vi "VI Tree.vi"   [LabVIEW 2022 SP3, in "Agilent ENA Series.lvlib"]
doc: "This is the instrument driver for the Agilent ENA Series RF Network Analyzer. The VI Tree displays all the user-callable VIs of the instrument driver in an organized table."
uses:
  <instrlib>/Agilent ENA Series/Agilent ENA Series.lvlib
panel:
  # "(c) 2005-2021 National Instruments.  ALL RIGHTS RESERVED."
  # "SEE DIAGRAM\nFOR VI TREE."
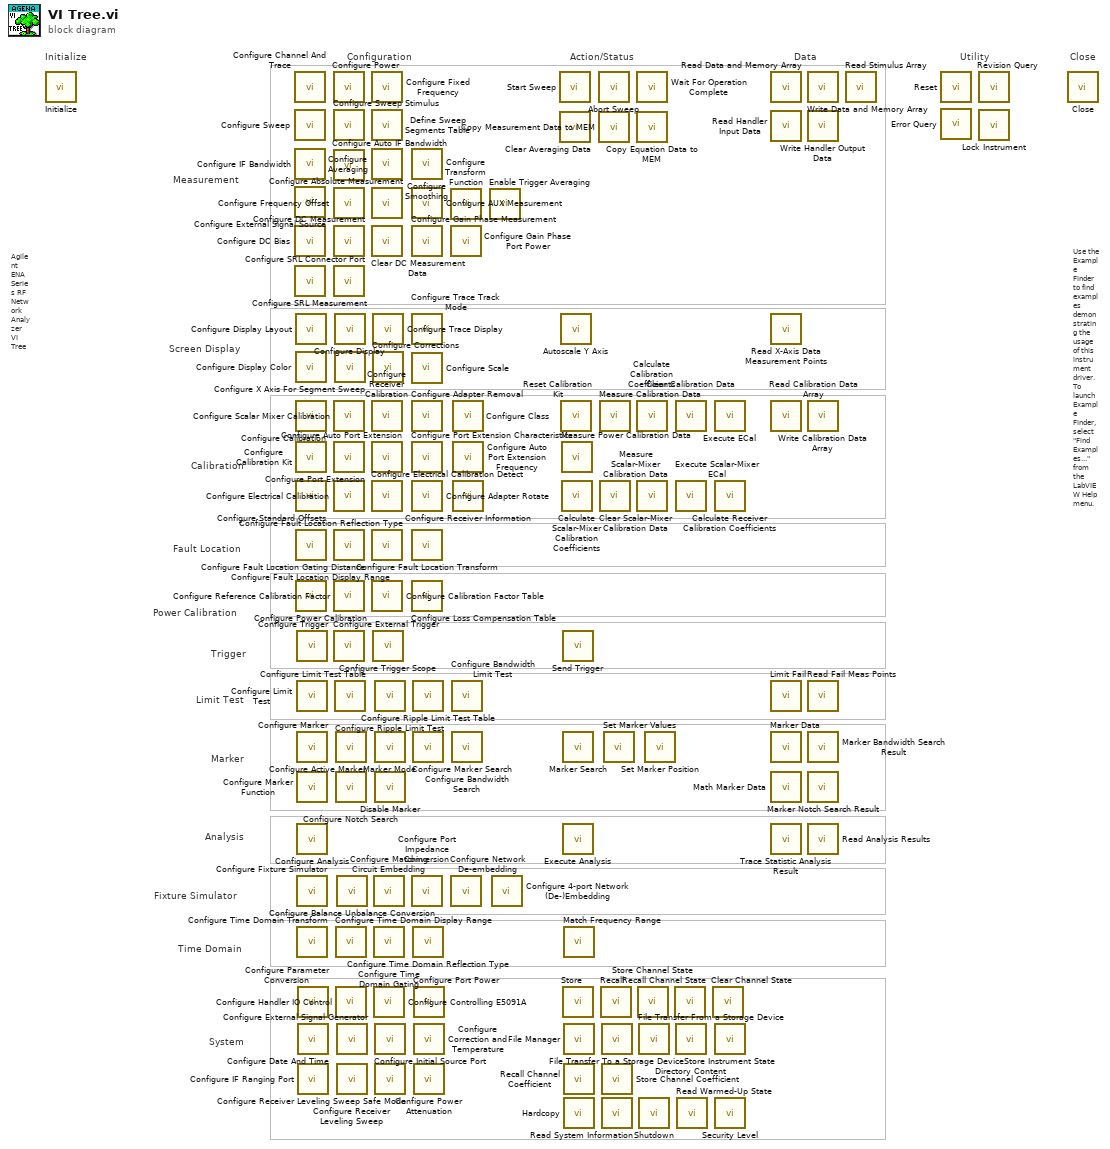
[diagram p0: block diagram]
diagram:
  # "Fault Location"
  # "Time Domain"
  # "System"
  # "Fixture Simulator"
  # "Analysis"
  # "Marker"
  # "Limit Test"
  # "Trigger"
  # "Power Calibration"
  # "Agilent ENA Series RF Network Analyzer VI Tree"
  # "Calibration"
  # "Screen Display"
  # "Measurement"
  # "Use the Example Finder to find examples demonstrating the usage of this instrument driver.\nTo launch Example Finder, select \"Find Examples...\" from the LabVIEW Help menu."
  # "Configuration"
  # "Utility"
  # "Data"
  # "Action/Status"
  # "Close"
  # "Initialize"
  n1 = call <instrlib>:"Initialize.vi"() -> ()  [unwired: 10 in, 2 out]
  n2 = call <instrlib>:"Configure Channel And Trace.vi"() -> ()  [unwired: 10 in, 2 out]
  n3 = call <instrlib>:"Configure Sweep.vi"() -> ()  [unwired: 14 in, 2 out]
  n4 = call <instrlib>:"Configure IF Bandwidth.vi"() -> ()  [unwired: 10 in, 2 out]
  n5 = call <instrlib>:"Configure External Signal Source.vi"() -> ()  [unwired: 18 in, 2 out]
  n6 = call <instrlib>:"Configure DC Bias.vi"() -> ()  [unwired: 10 in, 2 out]
  n7 = call <instrlib>:"Configure SRL Measurement.vi"() -> ()  [unwired: 10 in, 2 out]
  n8 = call <instrlib>:"Configure Display Layout.vi"() -> ()  [unwired: 10 in, 2 out]
  n9 = call <instrlib>:"Configure Display Color.vi"() -> ()  [unwired: 14 in, 2 out]
  n10 = call <instrlib>:"Configure Calibration.vi"() -> ()  [unwired: 18 in, 2 out]
  n11 = call <instrlib>:"Configure Calibration Kit.vi"() -> ()  [unwired: 26 in, 2 out]
  n12 = call <instrlib>:"Configure Standard Offsets.vi"() -> ()  [unwired: 10 in, 2 out]
  n13 = call <instrlib>:"Configure Fault Location Display Range.vi"() -> ()  [unwired: 14 in, 2 out]
  n14 = call <instrlib>:"Configure Power Calibration.vi"() -> ()  [unwired: 14 in, 2 out]
  n15 = call <instrlib>:"Configure Trigger.vi"() -> ()  [unwired: 10 in, 2 out]
  n16 = call <instrlib>:"Configure Limit Test.vi"() -> ()  [unwired: 10 in, 2 out]
  n17 = call <instrlib>:"Configure Marker.vi"() -> ()  [unwired: 10 in, 2 out]
  n18 = call <instrlib>:"Configure Marker Function.vi"() -> ()  [unwired: 10 in, 2 out]
  n19 = call <instrlib>:"Configure Analysis.vi"() -> ()  [unwired: 18 in, 2 out]
  n20 = call <instrlib>:"Configure Fixture Simulator.vi"() -> ()  [unwired: 14 in, 2 out]
  n21 = call <instrlib>:"Configure Time Domain Transform.vi"() -> ()  [unwired: 14 in, 2 out]
  n22 = call <instrlib>:"Configure Parameter Conversion.vi"() -> ()  [unwired: 14 in, 2 out]
  n23 = call <instrlib>:"Configure Date And Time.vi"() -> ()  [unwired: 14 in, 2 out]
  n24 = call <instrlib>:"Configure IF Ranging Port.vi"() -> ()  [unwired: 10 in, 2 out]
  n25 = call <instrlib>:"Configure Power.vi"() -> ()  [unwired: 14 in, 2 out]
  n26 = call <instrlib>:"Configure Sweep Stimulus.vi"() -> ()  [unwired: 10 in, 2 out]
  n27 = call <instrlib>:"Configure Auto IF Bandwidth.vi"() -> ()  [unwired: 10 in, 2 out]
  n28 = call <instrlib>:"Configure Frequency Offset.vi"() -> ()  [unwired: 18 in, 2 out]
  n29 = call <instrlib>:"Configure DC Measurement.vi"() -> ()  [unwired: 10 in, 2 out]
  n30 = call <instrlib>:"Configure SRL Connector Port.vi"() -> ()  [unwired: 10 in, 2 out]
  n31 = call <instrlib>:"Configure Scalar Mixer Calibration.vi"() -> ()  [unwired: 10 in, 2 out]
  n32 = call <instrlib>:"Configure Port Extension.vi"() -> ()  [unwired: 10 in, 2 out]
  n33 = call <instrlib>:"Configure Electrical Calibration.vi"() -> ()  [unwired: 10 in, 2 out]
  n34 = call <instrlib>:"Configure Fault Location Gating Distance.vi"() -> ()  [unwired: 14 in, 2 out]
  n35 = call <instrlib>:"Configure Reference Calibration Factor.vi"() -> ()  [unwired: 14 in, 2 out]
  n36 = call <instrlib>:"Configure External Trigger.vi"() -> ()  [unwired: 10 in, 2 out]
  n37 = call <instrlib>:"Configure Display.vi"() -> ()  [unwired: 26 in, 2 out]
  n38 = call <instrlib>:"Configure X Axis For Segment Sweep.vi"() -> ()  [unwired: 10 in, 2 out]
  n39 = call <instrlib>:"Configure Limit Test Table.vi"() -> ()  [unwired: 14 in, 2 out]
  n40 = call <instrlib>:"Configure Active Marker.vi"() -> ()  [unwired: 10 in, 2 out]
  n41 = call <instrlib>:"Configure Notch Search.vi"() -> ()  [unwired: 10 in, 2 out]
  n42 = call <instrlib>:"Configure Time Domain Display Range.vi"() -> ()  [unwired: 14 in, 2 out]
  n43 = call <instrlib>:"Configure Handler IO Control.vi"() -> ()  [unwired: 10 in, 2 out]
  n44 = call <instrlib>:"Configure Balance Unbalance Conversion.vi"() -> ()  [unwired: 14 in, 2 out]
  n45 = call <instrlib>:"Configure External Signal Generator.vi"() -> ()  [unwired: 14 in, 2 out]
  n46 = call <instrlib>:"Configure Receiver Leveling Sweep.vi"() -> ()  [unwired: 18 in, 2 out]
  n47 = call <instrlib>:"Configure Fixed Frequency.vi"() -> ()  [unwired: 10 in, 2 out]
  n48 = call <instrlib>:"Define Sweep Segments Table.vi"() -> ()  [unwired: 18 in, 2 out]
  n49 = call <instrlib>:"Configure Averaging.vi"() -> ()  [unwired: 10 in, 2 out]
  n50 = call <instrlib>:"Configure Absolute Measurement.vi"() -> ()  [unwired: 14 in, 2 out]
  n51 = call <instrlib>:"Clear DC Measurement Data.vi"() -> ()  [unwired: 10 in, 2 out]
  n52 = call <instrlib>:"Configure Receiver Calibration.vi"() -> ()  [unwired: 10 in, 2 out]
  n53 = call <instrlib>:"Configure Auto Port Extension.vi"() -> ()  [unwired: 10 in, 2 out]
  n54 = call <instrlib>:"Configure Electrical Calibration Detect.vi"() -> ()  [unwired: 10 in, 2 out]
  n55 = call <instrlib>:"Configure Fault Location Reflection Type.vi"() -> ()  [unwired: 10 in, 2 out]
  n56 = call <instrlib>:"Configure Calibration Factor Table.vi"() -> ()  [unwired: 10 in, 2 out]
  n57 = call <instrlib>:"Configure Trace Display.vi"() -> ()  [unwired: 14 in, 2 out]
  n58 = call <instrlib>:"Configure Corrections.vi"() -> ()  [unwired: 14 in, 2 out]
  n59 = call <instrlib>:"Configure Trigger Scope.vi"() -> ()  [unwired: 10 in, 2 out]
  n60 = call <instrlib>:"Configure Matching Circuit Embedding.vi"() -> ()  [unwired: 18 in, 2 out]
  n61 = call <instrlib>:"Configure Time Domain Gating.vi"() -> ()  [unwired: 14 in, 2 out]
  n62 = call <instrlib>:"Configure Controlling E5091A.vi"() -> ()  [unwired: 14 in, 2 out]
  n63 = call <instrlib>:"Configure Ripple Limit Test.vi"() -> ()  [unwired: 10 in, 2 out]
  n64 = call <instrlib>:"Marker Mode.vi"() -> ()  [unwired: 10 in, 2 out]
  n65 = call <instrlib>:"Disable Marker.vi"() -> ()  [unwired: 10 in, 2 out]
  n66 = call <instrlib>:"Configure Initial Source Port.vi"() -> ()  [unwired: 10 in, 2 out]
  n67 = call <instrlib>:"Configure Receiver Leveling Sweep Safe Mode.vi"() -> ()  [unwired: 10 in, 2 out]
  n68 = call <instrlib>:"Configure Smoothing.vi"() -> ()  [unwired: 10 in, 2 out]
  n69 = call <instrlib>:"Configure AUX Measurement.vi"() -> ()  [unwired: 14 in, 2 out]
  n70 = call <instrlib>:"Configure Gain Phase Measurement.vi"() -> ()  [unwired: 10 in, 2 out]
  n71 = call <instrlib>:"Configure Trace Track Mode.vi"() -> ()  [unwired: 10 in, 2 out]
  n72 = call <instrlib>:"Configure Scale.vi"() -> ()  [unwired: 14 in, 2 out]
  n73 = call <instrlib>:"Configure Adapter Removal.vi"() -> ()  [unwired: 10 in, 2 out]
  n74 = call <instrlib>:"Configure Port Extension Characteristics.vi"() -> ()  [unwired: 14 in, 2 out]
  n75 = call <instrlib>:"Configure Adapter Rotate.vi"() -> ()  [unwired: 10 in, 2 out]
  n76 = call <instrlib>:"Configure Fault Location Transform.vi"() -> ()  [unwired: 14 in, 2 out]
  n77 = call <instrlib>:"Configure Loss Compensation Table.vi"() -> ()  [unwired: 10 in, 2 out]
  n78 = call <instrlib>:"Configure Port Impedance Conversion.vi"() -> ()  [unwired: 14 in, 2 out]
  n79 = call <instrlib>:"Configure Ripple Limit Test Table.vi"() -> ()  [unwired: 14 in, 2 out]
  n80 = call <instrlib>:"Configure Marker Search.vi"() -> ()  [unwired: 18 in, 2 out]
  n81 = call <instrlib>:"Configure Time Domain Reflection Type.vi"() -> ()  [unwired: 10 in, 2 out]
  n82 = call <instrlib>:"Configure Port Power.vi"() -> ()  [unwired: 10 in, 2 out]
  n83 = call <instrlib>:"Configure Correction and Temperature.vi"() -> ()  [unwired: 10 in, 2 out]
  n84 = call <instrlib>:"Configure Power Attenuation.vi"() -> ()  [unwired: 10 in, 2 out]
  n85 = call <instrlib>:"Configure Transform Function.vi"() -> ()  [unwired: 10 in, 2 out]
  n86 = call <instrlib>:"Configure Gain Phase Port Power.vi"() -> ()  [unwired: 10 in, 2 out]
  n87 = call <instrlib>:"Configure Network De-embedding.vi"() -> ()  [unwired: 14 in, 2 out]
  n88 = call <instrlib>:"Configure Bandwidth Limit Test.vi"() -> ()  [unwired: 14 in, 2 out]
  n89 = call <instrlib>:"Configure Bandwidth Search.vi"() -> ()  [unwired: 10 in, 2 out]
  n90 = call <instrlib>:"Configure Class.vi"() -> ()  [unwired: 10 in, 2 out]
  n91 = call <instrlib>:"Configure Auto Port Extension Frequency.vi"() -> ()  [unwired: 14 in, 2 out]
  n92 = call <instrlib>:"Configure Receiver Information.vi"() -> ()  [unwired: 10 in, 2 out]
  n93 = call <instrlib>:"Enable Trigger Averaging.vi"() -> ()  [unwired: 10 in, 2 out]
  n94 = call <instrlib>:"Configure 4-port Network (De-)Embedding.vi"() -> ()  [unwired: 18 in, 2 out]
  n95 = call <instrlib>:"Start Sweep.vi"() -> ()  [unwired: 10 in, 2 out]
  n96 = call <instrlib>:"Clear Averaging Data.vi"() -> ()  [unwired: 10 in, 2 out]
  n97 = call <instrlib>:"Autoscale Y Axis.vi"() -> ()  [unwired: 10 in, 2 out]
  n98 = call <instrlib>:"Reset Calibration Kit.vi"() -> ()  [unwired: 10 in, 2 out]
  n99 = call <instrlib>:"Measure Power Calibration Data.vi"() -> ()  [unwired: 10 in, 2 out]
  n100 = call <instrlib>:"Calculate Scalar-Mixer Calibration Coefficients.vi"() -> ()  [unwired: 10 in, 2 out]
  n101 = call <instrlib>:"Send Trigger.vi"() -> ()  [unwired: 10 in, 2 out]
  n102 = call <instrlib>:"Marker Search.vi"() -> ()  [unwired: 7 in, 5 out]
  n103 = call <instrlib>:"Execute Analysis.vi"() -> ()  [unwired: 10 in, 2 out]
  n104 = call <instrlib>:"Store.vi"() -> ()  [unwired: 10 in, 2 out]
  n105 = call <instrlib>:"Match Frequency Range.vi"() -> ()  [unwired: 14 in, 2 out]
  n106 = call <instrlib>:"File Manager.vi"() -> ()  [unwired: 10 in, 2 out]
  n107 = call <instrlib>:"Recall Channel Coefficient.vi"() -> ()  [unwired: 10 in, 2 out]
  n108 = call <instrlib>:"Hardcopy.vi"() -> ()  [unwired: 10 in, 2 out]
  n109 = call <instrlib>:"Abort Sweep.vi"() -> ()  [unwired: 10 in, 2 out]
  n110 = call <instrlib>:"Copy Measurement Data to MEM.vi"() -> ()  [unwired: 10 in, 2 out]
  n111 = call <instrlib>:"Measure Calibration Data.vi"() -> ()  [unwired: 10 in, 2 out]
  n112 = call <instrlib>:"Clear Scalar-Mixer Calibration Data.vi"() -> ()  [unwired: 10 in, 2 out]
  n113 = call <instrlib>:"Recall.vi"() -> ()  [unwired: 10 in, 2 out]
  n114 = call <instrlib>:"File Transfer To a Storage Device.vi"() -> ()  [unwired: 10 in, 2 out]
  n115 = call <instrlib>:"Store Channel Coefficient.vi"() -> ()  [unwired: 10 in, 2 out]
  n116 = call <instrlib>:"Read System Information.vi"() -> ()  [unwired: 6 in, 6 out]
  n117 = call <instrlib>:"Set Marker Values.vi"() -> ()  [unwired: 10 in, 2 out]
  n118 = call <instrlib>:"Wait For Operation Complete.vi"() -> ()  [unwired: 10 in, 2 out]
  n119 = call <instrlib>:"Copy Equation Data to MEM.vi"() -> ()  [unwired: 10 in, 2 out]
  n120 = call <instrlib>:"Calculate Calibration Coefficients.vi"() -> ()  [unwired: 10 in, 2 out]
  n121 = call <instrlib>:"Measure Scalar-Mixer Calibration Data.vi"() -> ()  [unwired: 10 in, 2 out]
  n122 = call <instrlib>:"Store Channel State.vi"() -> ()  [unwired: 10 in, 2 out]
  n123 = call <instrlib>:"File Transfer From a Storage Device.vi"() -> ()  [unwired: 9 in, 3 out]
  n124 = call <instrlib>:"Shutdown.vi"() -> ()  [unwired: 10 in, 2 out]
  n125 = call <instrlib>:"Set Marker Position.vi"() -> ()  [unwired: 10 in, 2 out]
  n126 = call <instrlib>:"Recall Channel State.vi"() -> ()  [unwired: 10 in, 2 out]
  n127 = call <instrlib>:"Clear Calibration Data.vi"() -> ()  [unwired: 10 in, 2 out]
  n128 = call <instrlib>:"Execute Scalar-Mixer ECal.vi"() -> ()  [unwired: 10 in, 2 out]
  n129 = call <instrlib>:"Directory Content.vi"() -> ()  [unwired: 6 in, 6 out]
  n130 = call <instrlib>:"Read Warmed-Up State.vi"() -> ()  [unwired: 9 in, 3 out]
  n131 = call <instrlib>:"Clear Channel State.vi"() -> ()  [unwired: 10 in, 2 out]
  n132 = call <instrlib>:"Execute ECal.vi"() -> ()  [unwired: 10 in, 2 out]
  n133 = call <instrlib>:"Calculate Receiver Calibration Coefficients.vi"() -> ()  [unwired: 10 in, 2 out]
  n134 = call <instrlib>:"Store Instrument State.vi"() -> ()  [unwired: 10 in, 2 out]
  n135 = call <instrlib>:"Security Level.vi"() -> ()  [unwired: 10 in, 2 out]
  n136 = call <instrlib>:"Read Data and Memory Array.vi"() -> ()  [unwired: 8 in, 4 out]
  n137 = call <instrlib>:"Read Handler Input Data.vi"() -> ()  [unwired: 9 in, 3 out]
  n138 = call <instrlib>:"Read X-Axis Data Measurement Points.vi"() -> ()  [unwired: 9 in, 3 out]
  n139 = call <instrlib>:"Read Calibration Data Array.vi"() -> ()  [unwired: 9 in, 3 out]
  n140 = call <instrlib>:"Limit Fail.vi"() -> ()  [unwired: 9 in, 3 out]
  n141 = call <instrlib>:"Marker Data.vi"() -> ()  [unwired: 7 in, 5 out]
  n142 = call <instrlib>:"Math Marker Data.vi"() -> ()  [unwired: 6 in, 6 out]
  n143 = call <instrlib>:"Trace Statistic Analysis Result.vi"() -> ()  [unwired: 7 in, 5 out]
  n144 = call <instrlib>:"Write Data and Memory Array.vi"() -> ()  [unwired: 10 in, 2 out]
  n145 = call <instrlib>:"Write Handler Output Data.vi"() -> ()  [unwired: 10 in, 2 out]
  n146 = call <instrlib>:"Write Calibration Data Array.vi"() -> ()  [unwired: 10 in, 2 out]
  n147 = call <instrlib>:"Read Fail Meas Points.vi"() -> ()  [unwired: 8 in, 4 out]
  n148 = call <instrlib>:"Marker Bandwidth Search Result.vi"() -> ()  [unwired: 6 in, 6 out]
  n149 = call <instrlib>:"Marker Notch Search Result.vi"() -> ()  [unwired: 6 in, 6 out]
  n150 = call <instrlib>:"Read Analysis Results.vi"() -> ()  [unwired: 7 in, 5 out]
  n151 = call <instrlib>:"Read Stimulus Array.vi"() -> ()  [unwired: 9 in, 3 out]
  n152 = call <instrlib>:"Reset.vi"() -> ()  [unwired: 10 in, 2 out]
  n153 = call <instrlib>:"Error Query.vi"() -> ()  [unwired: 8 in, 4 out]
  n154 = call <instrlib>:"Revision Query.vi"() -> ()  [unwired: 8 in, 4 out]
  n155 = call <instrlib>:"Lock Instrument.vi"() -> ()  [unwired: 10 in, 2 out]
  n156 = call <instrlib>:"Close.vi"() -> ()  [unwired: 11 in, 1 out]
